vi "Belkin Demo Image Proc.vi"() -> ()   [LabVIEW 2015]
uses:
  <vilib>/userdefined/High Color/IMAQdx.ctl
  <vilib>/FPGAPlugInAG/cRIO-9030/niLvFpga_Open_cRIO-9030.vi
  <vilib>/rvi/interface/common/dynamic/niFpgaDynamicAddResources.vi
  <vilib>/Utility/error.llb/Error Cluster From Error Code.vi
  <vilib>/rvi/errors/niLvFpgaAdjustHostInterfaceError.vi
  <vilib>/FPGAPlugInAG/Dynamic/niLvFpga_Close_Dynamic.vi
  <vilib>/rvi/interface/nirviOpenFPGA/nirviOpenFPGA.xnode
  FPGA Bitfiles/BelkinDemo_FPGATarget_BelkinPolartoCom_2zVnbe-nqac.lvbitx
  FPGA/Belkin Polar to Complex.vi
  <vilib>/rvi/interface/nirviReadWriteControl/nirviReadWriteControl.xnode
  <vilib>/rvi/interface/nirviCloseFPGA/nirviCloseFPGA.xnode
  <vilib>/vision/NI_Vision_Development_Module.lvlib
  <vilib>/vision/driver/NI_Vision_Acquisition_Software.lvlib
  NiFpgaLv.dll
  <vilib>/rvi/interface/Simulation/niFpgaSimulationCallBeginRW.vi
panel:
  in  "Yofset":fxp<+/-,16,1>
  in  "Xofset":fxp<+/-,16,1>
  in  "Ygain":fxp<+/-,16,1>
  in  "Xgain":fxp<+/-,16,1>
  out "error out 3":errorcluster
  out "error out 2":errorcluster
  in  "Session In":T1
  out "Image Out":T2(plugin-control)
  in  "stop":bool
  out "Number of Matches Returned":i32
  out "Circles":T3(array[cluster])
  out "error out":errorcluster
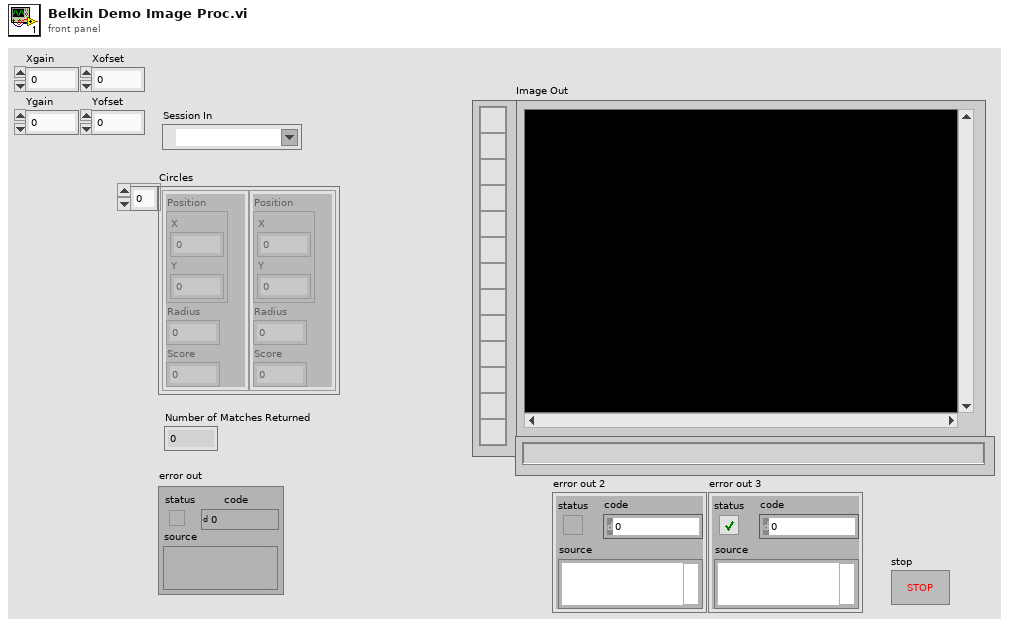
[diagram p1: front panel]
types:
  T1 = typedef "IMAQdx.ctl" = refnum<k21>
  T2 = typedef "IMAQ Image.ctl" = refnum<image>
  T3 = cluster{"Position":cluster{"X":sgl, "Y":sgl}, "Radius":dbl, "Score":dbl}[]
  T4 = typedef "Image Type" = u32
  T5 = cluster{"Extraction Mode":u32, "Edge Threshold":i32, "Edge Filter Size":u32, "Min Length":i32, "Row Search Step Size":i32, "Col Search Step Size":i32, "Max Endpoint Gap":i32, "Closed":bool, "Subpixel":bool}
  T6 = cluster{"Rotation":bool, "Scale":bool, "Occlusion":bool, "Range Settings":cluster{"Match Constraints":u32, "Min":dbl, "Max":dbl}[]}
  T7 = cluster{"Global Rectangle":i32[], "Contours":cluster{"ID":enum32{"External", "Internal"}, "Type":u32, "Coordinates":i32[]}[]}
  T8 = cluster{"Position":cluster{"X":sgl, "Y":sgl}, "Radius":dbl, "Score":dbl}
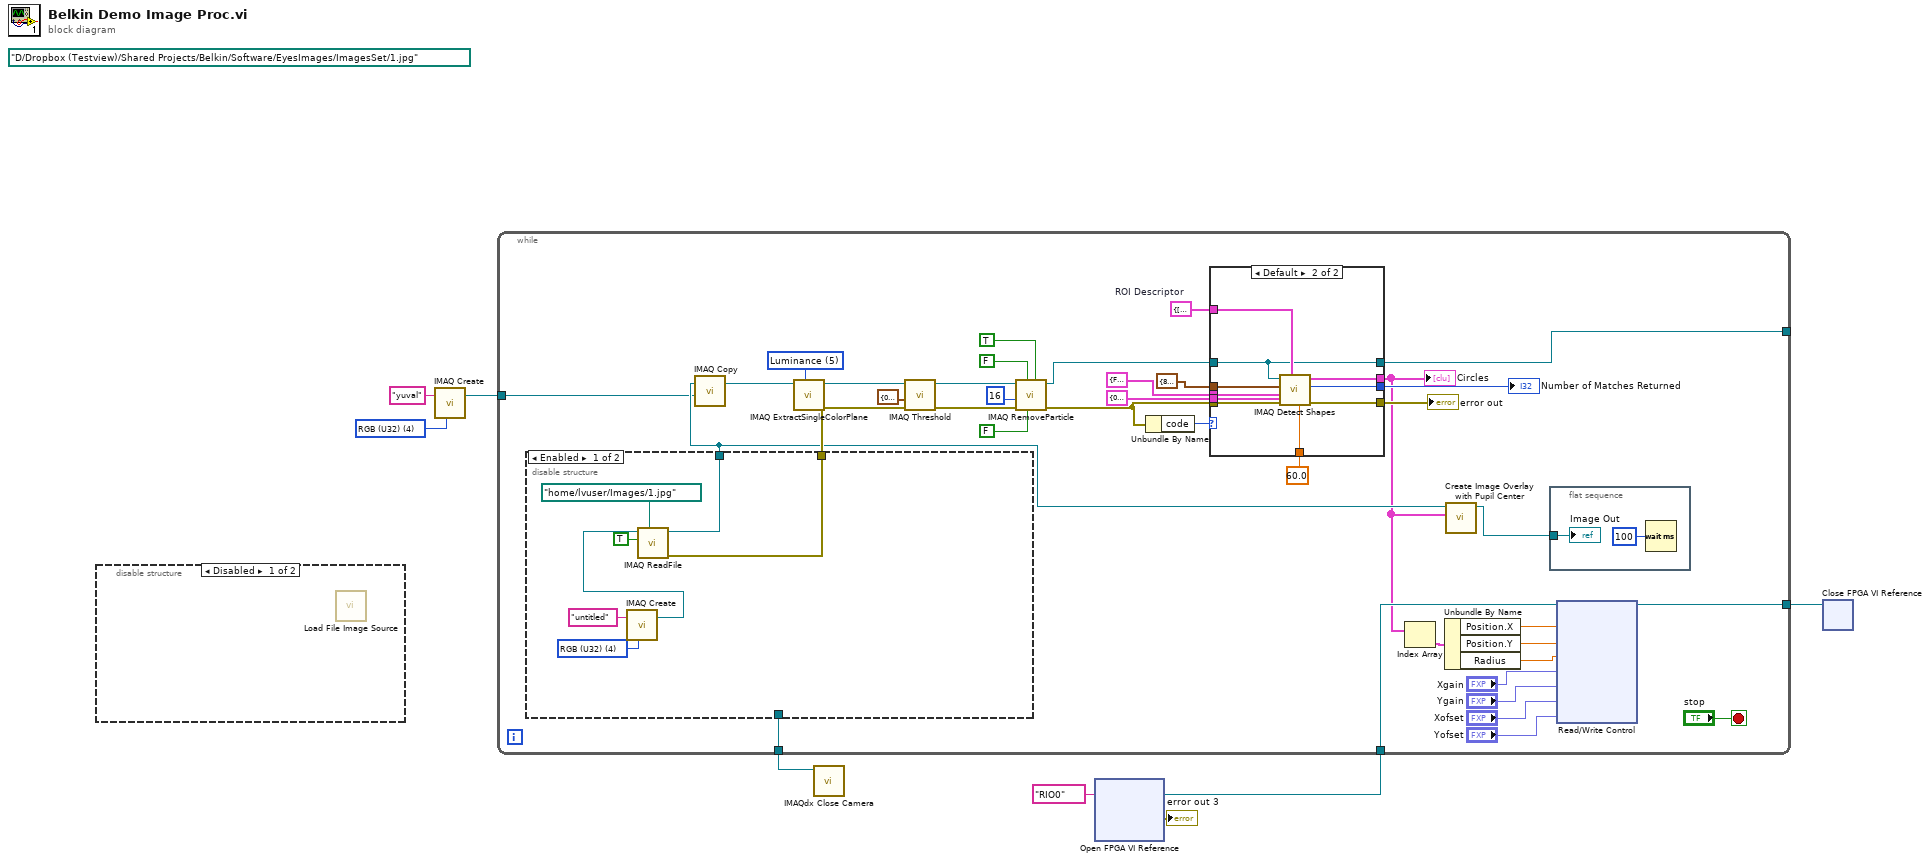
[diagram p0: block diagram]
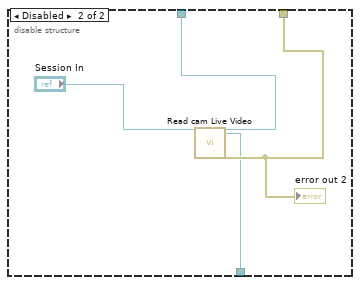
[diagram p2: hidden frame]
diagram:
  w7 = T4 4 items=["Grayscale (U8)", "Grayscale (I16)", "Grayscale (SGL)", "Complex (CSG)", "RGB (U32)", "HSL (U32)", "RGB (U64)", "Grayscale (U16)"] ("Image Type")
  (unwired) path "D:/Dropbox (Testview)/Shared Projects/Belkin/Software/EyesImages/ImagesSet/1.jpg" ("File Path")
  n1 = disable-structure shown="Disabled" {
    frame Disabled {
      n2 = call "Load File Image Source.vi"() -> ()  [unwired: 10 in, 2 out]
    }
    frame Enabled {
    }
  }
  n3 = call "IMAQ Create"("Image Name"="yuval", "Image Type"=w7) -> ("New Image"=w5:T2)  [unwired: 2 in, 2 out]
  n4 = xnode "Open FPGA VI Reference"("resource name"=tag "RIO0") -> ("FPGA VI Reference Out"=w3:refnum<k20>, "error out"=→"error out 3":errorcluster)  [unwired: 1 in]
  n5 = while {
    tunnel: [w22] -> _
    tunnel: [w21] -> w8
    tunnel: w5 -> [w20]
    tunnel: w3 -> [w19]
    tunnel: [w13] -> w2
    stop <- "stop" stop-if-true
    w32 = T7 {"Global Rectangle"=[14, 9, 1266, 998], "Contours"=[{"ID"=enum."External", "Type"=3, "Coordinates"=[14, 9, 1266, 998]}]}  # ROI Descriptor
    w47 = 5 items=["Red", "Green", "Blue", "Hue", "Saturation", "Luminance", "Value", "Intensity"] ("Color Plane")
    n6 = disable-structure shown="Enabled" {
      disable-tunnel: [w50 w58] -> w26
      disable-tunnel: [w48 w56] -> w23
      disable-tunnel: [_ w55] -> w21
      frame Enabled {
        w49 = T4 4 items=["Grayscale (U8)", "Grayscale (I16)", "Grayscale (SGL)", "Complex (CSG)", "RGB (U32)", "HSL (U32)", "RGB (U64)", "Grayscale (U16)"] ("Image Type")
        n7 = call "IMAQ Create"("Image Name"="untitled", "Image Type"=w49) -> ("New Image"=w51:T2)  [unwired: 2 in, 2 out]
        n8 = call "IMAQ ReadFile"("File Path"=path "/home/lvuser/Images/1.jpg", "Load Color Palette? (No)"=TRUE, "Image"=w51) -> ("error out"=w50:errorcluster, "Image Out"=w48:T2)  [unwired: 4 in, 3 out]
      }
      frame Disabled {
        n9 = call "Read cam Live Video.vi"("Session In"="Session In") -> ("Image Out"=w56:T2, "Session Out"=w55:T1, "error out"=w58:errorcluster)  [unwired: 24 in]
        "error out 2" <- w58
      }
    }
    n10 = call "IMAQ Copy"("Image Dst"=w20, "Image Src"=w23) -> ("Image Dst Out"=w24:T2)  [unwired: 1 in, 4 out]
    n11 = call "IMAQ ExtractSingleColorPlane"("Color Plane"=w47, "error in (no error)"=w26, "Image Src"=w24) -> ("error out"=w46:errorcluster, "Image Dst Out"=w44:T2)  [unwired: 1 in, 6 out]
    n12 = call "IMAQ Threshold"("error in (no error)"=w46, "Range"=cluster{"Lower value":sgl, "Upper value":sgl} {"Lower value"=0.0, "Upper value"=47.0}, "Image Src"=w44) -> ("error out"=w43:errorcluster, "Image Dst Out"=w38:T2)  [unwired: 3 in, 4 out]
    n13 = call "IMAQ RemoveParticle"("Connectivity 4/8 (8)"=TRUE, "Low Pass/High Pass (Low)"=FALSE, "Square/Hexa (Square)"=FALSE, "error in (no error)"=w43, "Number of Erosion"=16, "Image Src"=w38) -> ("error out"=w37:errorcluster, "Image Dst Out"=w31:T2)  [unwired: 1 in, 3 out]
    n14 = Unbundle By Name(w37) -> ("code"=w30:i32)
    n15 = case shown="Default" w30 {
      tunnel: w37 -> [_ w71]
      tunnel: [_ w70] -> w28
      tunnel: T6 {"Rotation"=FALSE, "Scale"=FALSE, "Occlusion"=TRUE, "Range Settings"=[{"Match Constraints"=2, "Min"=0.0, "Max"=50.0}]} ("Match Options") -> [_ w69]
      tunnel: T5 {"Extraction Mode"=0, "Edge Threshold"=1, "Edge Filter Size"=1, "Min Length"=40, "Row Search Step Size"=61, "Col Search Step Size"=61, "Max Endpoint Gap"=10, "Closed"=FALSE, "Subpixel"=FALSE} ("Curve Parameters") -> [_ w68]
      tunnel: 60.0 ("Minimum match score") -> [_ w67]
      tunnel: cluster{"Min Radius":dbl, "Max Radius":dbl} {"Min Radius"=80.0, "Max Radius"=500.0} ("Circle Descriptor") -> [_ w66]
      tunnel: w32 -> [_ w65]
      tunnel: [_ w64] -> w18
      tunnel: w31 -> [w61 w62]
      tunnel: [_ w63] -> w29
      tunnel: [w61 w62] -> w22
      frame -1074396199, -1074396198 {
        # "Discard Coordinate\nSystem Error"
      }
      frame Default {
        n16 = call-poly "IMAQ Detect Shapes"("Minimum match score"=w67, "Curve Parameters"=w68, "ROI Descriptor"=w65, "error in (no error)"=w71, "Match Options"=w69, "Circle Descriptor"=w66, "Image"=w62) -> ("error out"=w63:errorcluster, "Number of Matches Returned"=w70:i32, "Circles"=w64:T3)  [unwired: 2 out]
      }
    }
    "error out" <- w29
    "Circles" <- w18
    "Number of Matches Returned" <- w28
    n17 = Index Array(array=w18) -> (element=w17:T8)  [unwired: 1 in]
    n18 = Unbundle By Name(w17) -> ("Position.X"=w16:sgl, "Position.Y"=w15:sgl, "Radius"=w14:dbl)
    n19 = call "Create Image Overlay with Pupil Center.vi"("Circles"=w18, "Refnum in"=w23) -> ("Refnum out"=w25:T2)  [unwired: 9 in]
    n20 = flat-sequence {
      tunnel: w25 -> [w60]
      frame #0 {
        n21 = Wait (ms)(milliseconds to wait=u32 100) -> ()  [unwired: 1 out]
        "Image Out" <- w60
      }
    }
    n22 = xnode "Read/Write Control"("FPGA VI Reference In"=w19, "Xpos"=w16, "Ypos"=w15, "PupilRadius"=w14, "Xgain"="Xgain", "Ygain"="Ygain", "Xofset"="Xofset", "Yofset"="Yofset") -> ("FPGA VI Reference Out"=w13:refnum<k20>)  [unwired: 1 in, 1 out]
  }
  n23 = call <vilib>:"IMAQdx Close Camera.vi"("Session In"=w8) -> ()  [unwired: 1 in, 10 out]
  n24 = xnode "Close FPGA VI Reference"("FPGA VI Reference In"=w2) -> ()  [unwired: 1 in, 1 out]
